vi "Create_setup_string.vi"() -> (0 "Setup String":string)   [LabVIEW 2010]
uses:
  Globals/Meas_global.vi
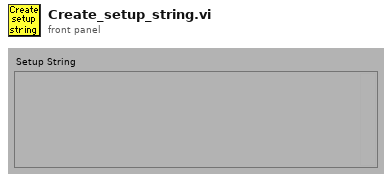
[diagram p1: front panel]
types:
  T1 = typedef "Analysis_info_cluster.ctl" = cluster{"Colour":u32, "Inst type":T2, "Inst name":string, "Symbol":string, "Code name":string, "Extra Info":string, "Inst Array":T3, "Index":i32, "Voltage Index":i32, "Extra Titles":string[], "Extra Values":string[]}
  T2 = typedef "Inst_type.ctl" = enum16{"Propeller anemometer", "Raw voltage", "Pressure Transducer", "Pitot-static tube", "Preston tube", "Hot wire", "Cross wire 1", "Cross wire 2", "Generic Linear", "Generic Polynomial", "Generic BackPoly", "Fast FID", "Thermocouple", "Cold wire", "Pulsed Wire", "LDA Vel", "LDA Tran time", "LDA Arr time"}
  T3 = typedef "Instrument_Array.ctl" = enum16{"PWA", "LDA", "Analogue"}
  T4 = typedef "Ch_and_Spans.ctl" = cluster{"high limit (10V)":sgl, "low limit (-10V)":sgl, "Ch No":i16, "Var name":string, "Use Latest Calib":bool}
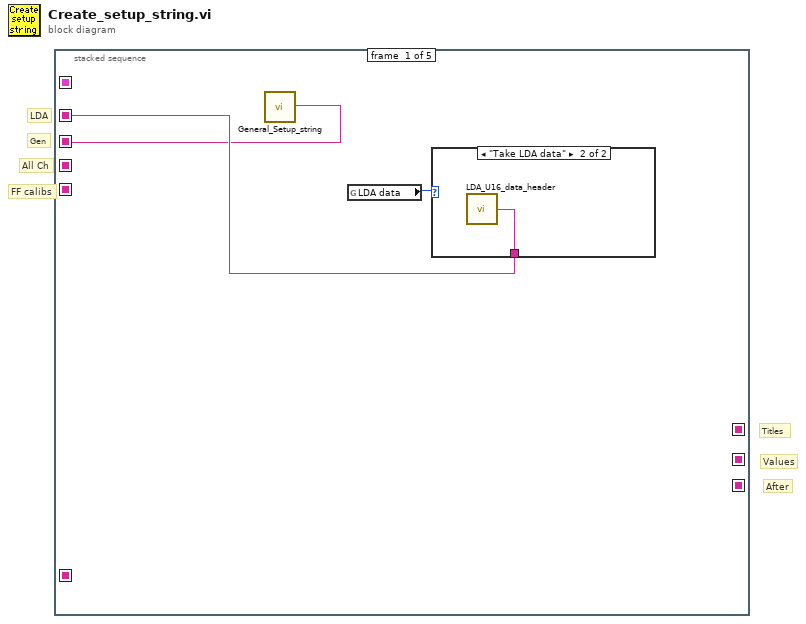
[diagram p0: block diagram]
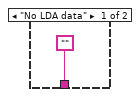
[diagram p2: hidden frame]
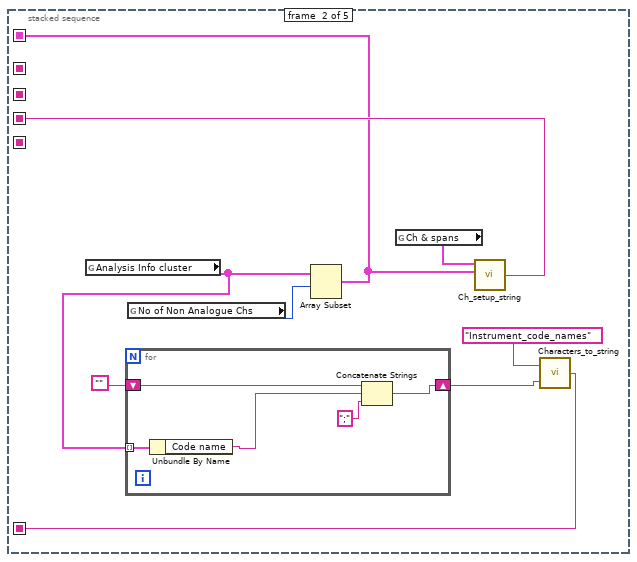
[diagram p3: hidden frame]
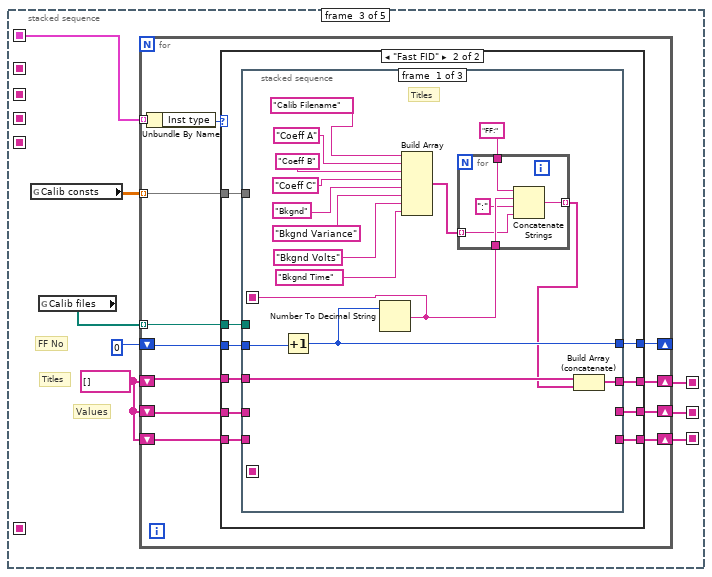
[diagram p4: hidden frame]
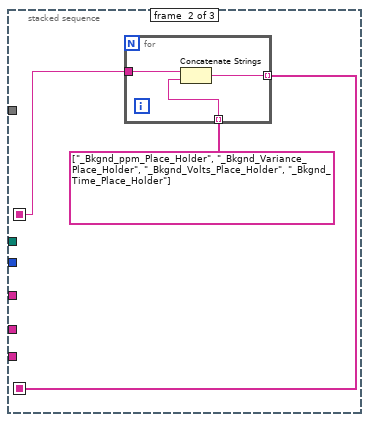
[diagram p6: hidden frame]
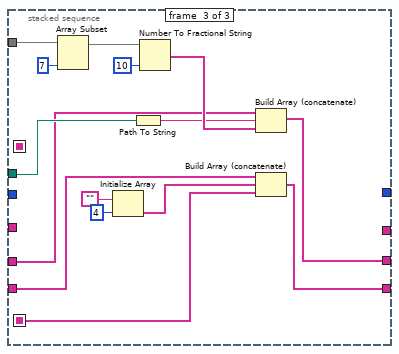
[diagram p7: hidden frame]
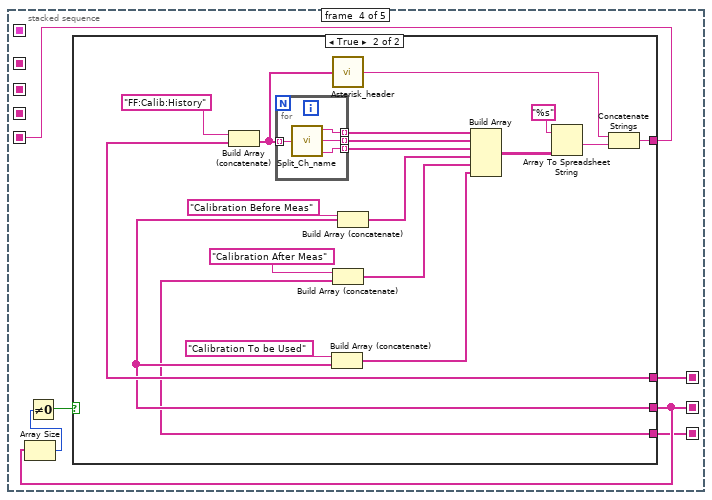
[diagram p8: hidden frame]
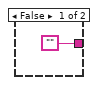
[diagram p9: hidden frame]
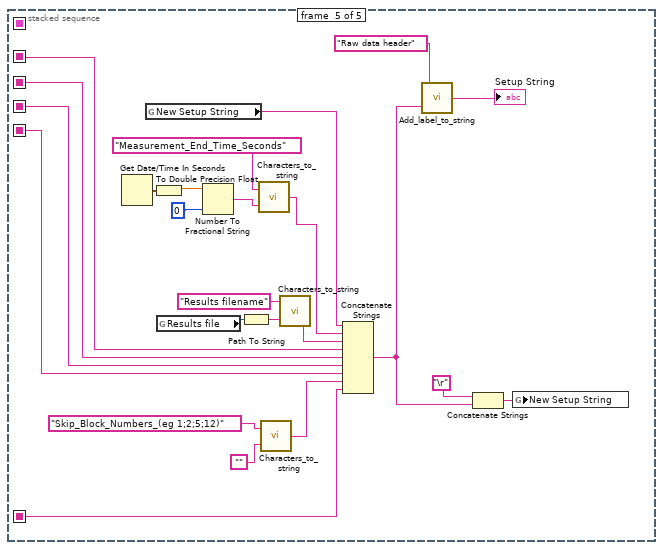
[diagram p10: hidden frame]
diagram:
  # "After"
  # "Values"
  # "Titles"
  # "FF calibs"
  # "LDA"
  # "Gen"
  # "All Ch"
  n1 = stacked-sequence {
    seq-local: [w3 _ _ _ _] -> [_ _ _ _ w149]
    seq-local: [w1 _ _ _ _] -> [_ _ _ _ w148]
    seq-local: [_ w14 _ _ _] -> [_ _ _ _ w147]
    seq-local: [_ _ _ w100 _] -> [_ _ _ _ w141]
    seq-local: [_ _ w23 _ _] -> [_ _ _ w101 _]
    seq-local: [_ _ w24 _ _] -> [_ _ _ w98 _]
    seq-local: [_ w12 _ _ _] -> [_ _ w22 _ _]
    seq-local: [_ _ w20 _ _] -> [_ _ _ w96 _]
    seq-local: [_ w6 _ _ _] -> [_ _ _ _ w126]
    frame #0 {
      n2 = call "General_Setup_string.vi"() -> ("Output string"=w1:string)  [unwired: 1 out]
      n3 = global read "Meas_global.vi" "LDA data"() -> (w2:enum16{"No LDA data", "Take LDA data"})
      n4 = case shown="\"Take LDA data\"" w2 {
        tunnel: ["" w5] -> w3
        frame "No LDA data" {
        }
        frame "Take LDA data" {
          n5 = call "LDA_U16_data_header.vi"() -> ("Output string"=w5:string)  [unwired: 1 out]
        }
      }
    }
    frame #1 {
      n6 = global read "Meas_global.vi" "Analysis Info cluster"() -> (w10:T1[])
      n7 = for {
        tunnel: w10 -> [w19] mode=indexing
        shift-right: [w15] -> w8
        shift-left: "" -> [w18]
        n8 = Unbundle By Name(w19) -> ("Code name"=w17:string)
        n9 = Concatenate Strings(w18, w17, ";" ("string")) -> (w15:string)
      }
      n10 = global read "Meas_global.vi" "No of Non Analogue Chs"() -> (w13:i32)
      n11 = Array Subset(array=w10, index=w13) -> (w12:T1[])  [unwired: 1 in]
      n12 = global read "Meas_global.vi" "Ch & spans"() -> (w11:T4[])
      n13 = call "Ch_setup_string.vi"("Analysis Info cluster (An Chs)"=w12, "Ch & spans"=w11) -> ("Output string"=w14:string)  [unwired: 1 in, 3 out]
      n14 = call "Characters_to_string.vi"("Characters to write"=w8, "Label for characters"="Instrument_code_names") -> ("Output string"=w6:string)
    }
    frame #2 {
      w21 = string[] []
      # "Values"
      # "Titles"
      # "FF No"
      n15 = global read "Meas_global.vi" "Calib consts"() -> (w27:dbl[][])
      n16 = global read "Meas_global.vi" "Calib files"() -> (w26:path[])
      n17 = for {
        tunnel: w22 -> [w39] mode=indexing
        tunnel: w27 -> [w37] mode=indexing
        tunnel: w26 -> [w36] mode=indexing
        shift-right: [w32] -> w23
        shift-left: w21 -> [w33]
        shift-right: [w34] -> _
        shift-left: 0 -> [w35]
        shift-right: [w30] -> w24
        shift-left: w21 -> [w31]
        shift-right: [w28] -> w20
        shift-left: w21 -> [w29]
        n18 = Unbundle By Name(w39) -> ("Inst type"=w38:T2)
        n19 = case shown="\"Fast FID\"" w38 {
          tunnel: w37 -> [_ w53]
          tunnel: w36 -> [_ w52]
          tunnel: w35 -> [w43 w51]
          tunnel: [w43 w50] -> w34
          tunnel: w33 -> [w42 w49]
          tunnel: [w42 w48] -> w32
          tunnel: w31 -> [w41 w47]
          tunnel: [w41 w46] -> w30
          tunnel: w29 -> [w40 w45]
          tunnel: [w40 w44] -> w28
          frame "Propeller anemometer", Default {
          }
          frame "Fast FID" {
            n20 = stacked-sequence {
              seq-local: [w54 _ _] -> [_ w76 _]
              seq-local: [_ w75 _] -> [_ _ w81]
              tunnel: w53 -> [_ _ w94]
              tunnel: w52 -> [_ _ w95]
              tunnel: w51 -> [w69 _ _]
              tunnel: [w66 _ _] -> w50
              tunnel: w49 -> [w64 _ _]
              tunnel: [w63 _ _] -> w48
              tunnel: w47 -> [_ _ w89]
              tunnel: [_ _ w88] -> w46
              tunnel: w45 -> [_ _ w86]
              tunnel: [_ _ w85] -> w44
              frame #0 {
                # "Titles"
                n21 = Increment(x=w69) -> (x+1=w66:i32)
                n22 = Number To Decimal String(number=w66) -> (decimal integer string=w54:string)  [unwired: 1 out]
                n23 = Build Array("Calib Filename", "Coeff A", "Coeff B", "Coeff C", "Bkgnd", "Bkgnd Variance", "Bkgnd Volts", "Bkgnd Time") -> (w65:string[])
                n24 = for {
                  tunnel: "FF:" -> [w74]
                  tunnel: w54 -> [w73]
                  tunnel: w65 -> [w71] mode=indexing
                  tunnel: [w70] -> w57 mode=indexing
                  n25 = Concatenate Strings(w74, w73, ":" ("Substring"), w71) -> (w70:string)
                }
                n26 = Build Array (concatenate)(w64, w57) -> (w63:string[])
              }
              frame #1 {
                n27 = for {
                  tunnel: string[] ["_Bkgnd_ppm_Place_Holder", "_Bkgnd_Variance_Place_Holder", "_Bkgnd_Volts_Place_Holder", "_Bkgnd_Time_Place_Holder"] -> [w80] mode=indexing
                  tunnel: w76 -> [w79]
                  tunnel: [w78] -> w75 mode=indexing
                  n28 = Concatenate Strings(w79, w80) -> (w78:string)
                }
              }
              frame #2 {
                n29 = Array Subset(array=w94, length=7 ("Array Length")) -> (w92:dbl[])  [unwired: 1 in]
                n30 = Initialize Array("", 4 ("dimension size")) -> (w82:string[])
                n31 = Path To String(path=w95) -> (string=w87:string)
                n32 = Number To Fractional String(number=w92, precision (6)=i16 10) -> (F-format string=w90:string[])  [unwired: 2 out]
                n33 = Build Array (concatenate)(w89, w87, w90) -> (w88:string[])
                n34 = Build Array (concatenate)(w86, w82, w81) -> (w85:string[])
              }
            }
          }
        }
      }
    }
    frame #3 {
      n35 = Array Size(array=w98) -> (size(s)=w99:i32)
      n36 = Not Equal To 0?(x=w99) -> (x != 0?=w97:bool)
      n37 = case shown="True" w97 {
        tunnel: w101 -> [_ w118]
        tunnel: w98 -> [_ w112]
        tunnel: ["" w106] -> w100
        tunnel: w96 -> [_ w104]
        frame False {
        }
        frame True {
          n38 = Build Array (concatenate)("FF:Calib:History" ("Input Element"), w118) -> (w109:string[])
          n39 = for {
            tunnel: w109 -> [w125] mode=indexing
            tunnel: [w124] -> w121 mode=indexing
            tunnel: [w123] -> w120 mode=indexing
            tunnel: [w122] -> w119 mode=indexing
            n40 = call "Split_Ch_name.vi"("Ch name"=w125) -> ("Top level"=w124:string, "Middle"=w123:string, "Low level"=w122:string)
          }
          n41 = Build Array (concatenate)("Calibration To be Used" ("Input Element"), w112) -> (w114:string[])
          n42 = call "Asterisk_header.vi"("Channel names"=w109) -> ("Header string"=w107:string)
          n43 = Build Array (concatenate)("Calibration After Meas" ("Input Element"), w104) -> (w103:string[])
          n44 = Build Array (concatenate)("Calibration Before Meas" ("Input Element"), w112) -> (w115:string[])
          n45 = Build Array(w121, w120, w119, w115, w103, w114) -> (w110:string[][])
          n46 = Array To Spreadsheet String(array=w110, 3:"%s" ("format string")) -> (spreadsheet string=w108:string)  [unwired: 1 out]
          n47 = Concatenate Strings(w107, w108) -> (w106:string)
        }
      }
    }
    frame #4 {
      n48 = Get Date/Time In Seconds() -> (seconds since 1Jan1904=w133:timestamp)
      n49 = global read "Meas_global.vi" "New Setup String"() -> (w136:string)
      n50 = To Double Precision Float(number=w133) -> (double precision float=w135:dbl)
      n51 = global read "Meas_global.vi" "Results file"() -> (w144:path)
      n52 = Number To Fractional String(number=w135, precision (6)=i16 0) -> (F-format string=w132:string)  [unwired: 2 out]
      n53 = Path To String(path=w144) -> (string=w140:string)
      n54 = call "Characters_to_string.vi"("Characters to write"=w132, "Label for characters"="Measurement_End_Time_Seconds") -> ("Output string"=w130:string)
      n55 = call "Characters_to_string.vi"("Characters to write"="", "Label for characters"="Skip_Block_Numbers_(eg 1;2;5;12)" ("Variable name")) -> ("Output string"=w127:string)
      n56 = call "Characters_to_string.vi"("Characters to write"=w140, "Label for characters"="Results filename") -> ("Output string"=w145:string)
      n57 = Concatenate Strings(w136, w130, w145, w149, w148, w147, w141, w127, w126) -> (w138:string)
      n58 = call "Add_label_to_string.vi"("String to write"=w138, "File Label"="Raw data header") -> ("Output string"=→"Setup String":string)
      n59 = Concatenate Strings("\r", w138) -> (w139:string)
      n60 = global write "Meas_global.vi" "New Setup String"(w139) -> ()
    }
  }
